vi "LSCI 370 Data Sensor.vi"(0 "VISA session":refnum<visa-resource-name>, 7 "Channel (1)":u16(ring)=1 items=["A", "1", "2", "3", "4", "5", "6", "7", "8", "9", "10", "11", "12", "13", "14", "15", "16"], 11 "error in (no error)":errorcluster) -> (4 "dup VISA session":refnum<visa-resource-name>, 6 "Resistance Reading":dbl min=0.0 max=63200000.0 step=1e-05 format="%^.5e", 8 "Kelvin Reading":dbl min=0.0 max=1000.0 step=1e-05 format="%^.5e", 10 "Power Reading":dbl min=0.0 max=0.01 step=1e-05 format="%^.5e", 15 "error out":errorcluster)   [LabVIEW 2016]
doc: "This VI querys the instrument for an channels's sensor reading in Resistance, Kelvin, and Power."
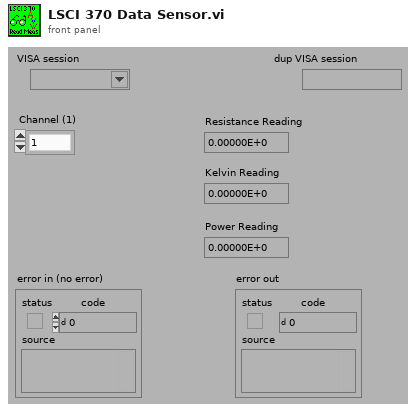
[diagram p1: front panel]
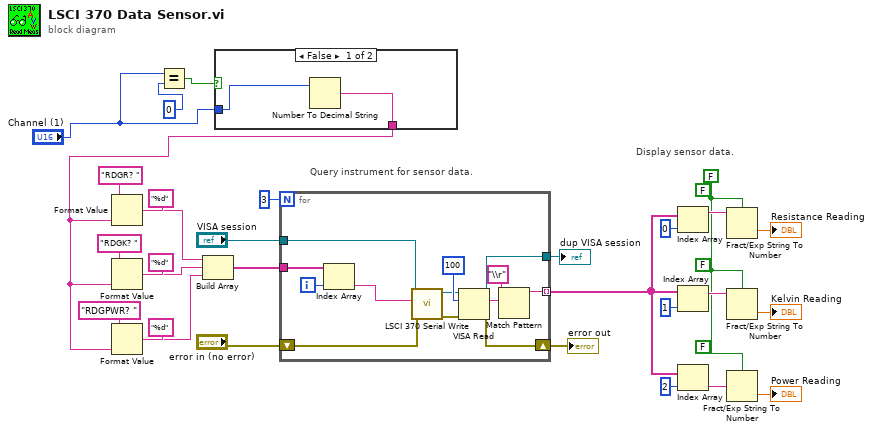
[diagram p0: block diagram]
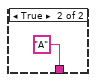
[diagram p2: hidden frame]
diagram:
  (unwired) FALSE ("use system decimal point (T)")
  (unwired) FALSE ("use system decimal point (T)")
  (unwired) FALSE ("use system decimal point (T)")
  w17 = FALSE ("use system decimal point (T)")
  # "Query instrument for sensor data."
  # "Display sensor data."
  n1 = Equal?(x="Channel (1)", y=0) -> (x = y?=w3:bool)
  n2 = case shown="False" w3 {
    tunnel: [w32 "A"] -> w1
    tunnel: "Channel (1)" -> [w31 _]
    frame False {
      n3 = Number To Decimal String(number=w31) -> (decimal integer string=w32:string)  [unwired: 1 in]
    }
    frame True {
    }
  }
  n4 = Format Value(string ("")="RDGR? ", format string="%d", value (0)=w1) -> (output string=w10:string)
  n5 = Format Value(string ("")="RDGK? ", format string="%d", value (0)=w1) -> (output string=w9:string)
  n6 = Format Value(string ("")="RDGPWR? ", format string="%d", value (0)=w1) -> (output string=w8:string)
  n7 = Build Array(w10, w9, w8) -> (w24:string[])
  n8 = for {
    N: 3 -> [_]
    tunnel: w24 -> [w43]
    shift-right: [w40] -> w20
    shift-left: "error in (no error)" -> [w41]
    tunnel: [w39] -> w19
    tunnel: "VISA session" -> [w38]
    tunnel: [w36] -> w18 mode=indexing
    i -> [w42]
    n9 = Index Array(array=w43, index=w42) -> (element=w34:string)
    n10 = call "LSCI 370 Serial Write.vi"("error in (no error)"=w41, "Write Buffer (\"\")"=w34, "VISA session"=w38) -> ("error out"=w46:errorcluster, "dup VISA session"=w35:refnum<visa-resource-name>)  [unwired: 6 in, 1 out]
    n11 = VISA Read(VISA resource name=w35, byte count=100, error in (no error)=w46) -> (VISA resource name out=w39:refnum<visa-resource-name>, read buffer=w44:string, error out=w40:errorcluster)  [unwired: 1 out]
    n12 = Match Pattern(string=w44, regular expression="\\r") -> (before substring=w36:string)  [unwired: 1 in, 3 out]
  }
  "dup VISA session" <- w19
  "error out" <- w20
  n13 = Index Array(array=w18, index=0) -> (element=w28:string)
  n14 = Index Array(array=w18, index=1) -> (element=w29:string)
  n15 = Index Array(array=w18, index=2) -> (element=w30:string)
  n16 = Fract/Exp String To Number(use system decimal point (T)=w17, string=w28) -> (number=→"Resistance Reading":dbl)  [unwired: 2 in, 1 out]
  n17 = Fract/Exp String To Number(use system decimal point (T)=w17, string=w29) -> (number=→"Kelvin Reading":dbl)  [unwired: 2 in, 1 out]
  n18 = Fract/Exp String To Number(use system decimal point (T)=w17, string=w30) -> (number=→"Power Reading":dbl)  [unwired: 2 in, 1 out]
